vi "gaussian (SubVI).vi"(6 "sigma":dbl, 9 "kernel":i32, 10 "Image Pixels (I16)":i16[][](array[numeric]), 11 "Iteratons number":dbl) -> (3 "imageOUT":u16[][](array[numeric]))   [LabVIEW 2016]
uses:
  Gauss.dll
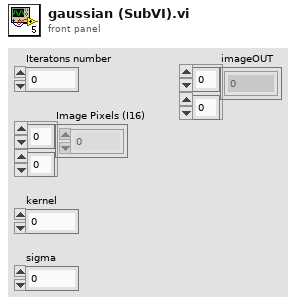
[diagram p1: front panel]
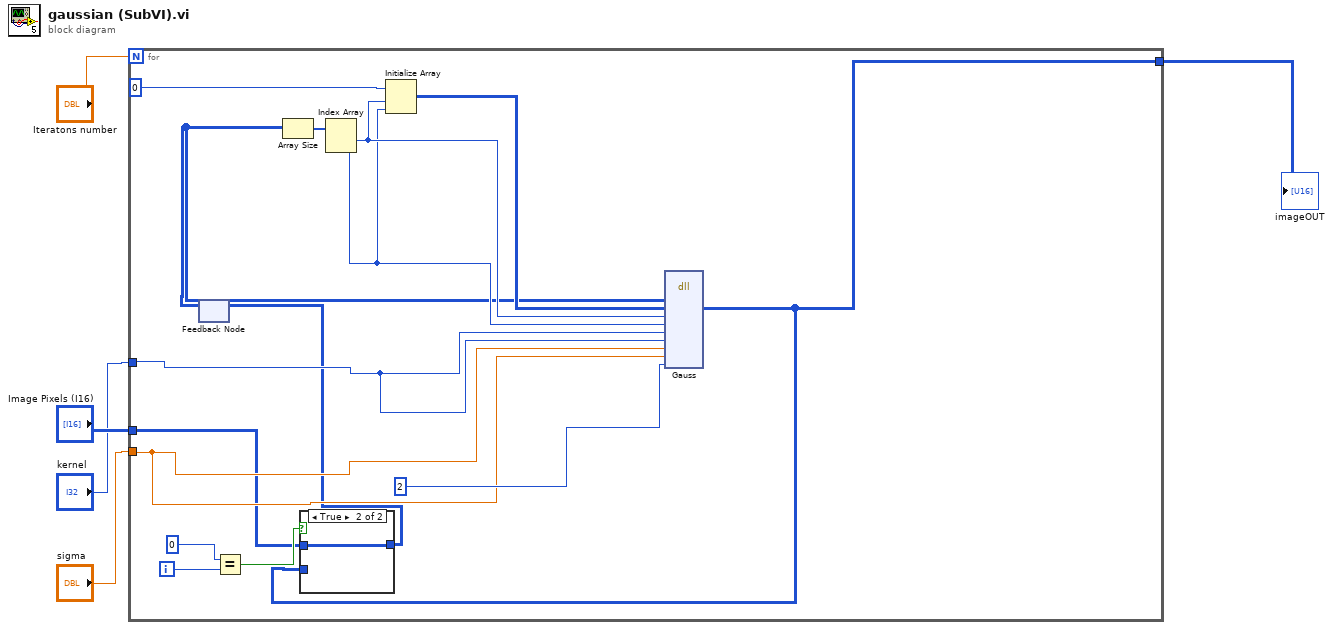
[diagram p0: block diagram]
diagram:
  n1 = for {
    N: "Iteratons number" -> [_]
    tunnel: [w8] -> w1
    tunnel: "kernel" -> [w14]
    tunnel: "sigma" -> [w13]
    tunnel: "Image Pixels (I16)" -> [w9]
    i -> [w12]
    n2 = feedback #1() -> (w6:u16[][])  [unwired: 1 in]
    n3 = Equal?(x=0, y=w12) -> (x = y?=w10:bool)
    n4 = Array Size(array=w6) -> (size(s)=w17:i32[])
    n5 = Index Array(array=w17) -> (element #1=w16:i32, element #2=w15:i32)  [unwired: 2 in]
    n6 = Initialize Array(u8 0 ("element"), w16, w15) -> (w19:u8[][])
    n7 = dll-call lib="G:/bsuir/mag/prytkov/GaussianImageProcessor/Gauss.dll" fn="Gauss"("imageIN"=w6, "imageOUT"=w19, "rows"=w16, "cols"=w15, "kernelX"=w14, "kernelY"=w14, "sigmaX"=w13, "sigmaY"=w13, "borderType"=2) -> ("imageOUT"=w8:u16[][])  [unwired: 12 in, 2 out]
    n8 = case shown="True" w10 {
      tunnel: [w21 w22] -> w7
      tunnel: w9 -> [_ w22]
      tunnel: w8 -> [w21 _]
      frame False {
      }
      frame True {
      }
    }
    n9 = feedback-in #1(w7) -> ()
  }
  "imageOUT" <- w1
